vi "_Read Sever Control.vi"(4 "error in (no error)":errorcluster, 5 "Text? (F)":bool, 7 "Control Ref":refnum<vi>) -> (0 "error out":errorcluster, 1 "Text":string, 2 "Boolean":bool)   [LabVIEW 2012]
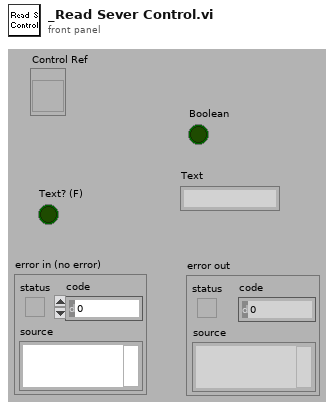
[diagram p1: front panel]
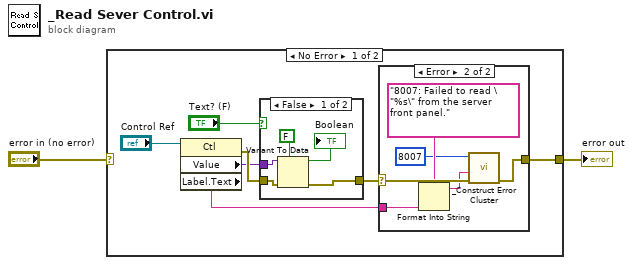
[diagram p0: block diagram]
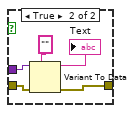
[diagram p3: hidden frame]
diagram:
  n1 = case shown="No Error" "error in (no error)" {
    selector: "error in (no error)" -> [_ w26]
    tunnel: [w9 w26] -> w1
    frame No Error {
      n2 = property class="Ctl"(reference="Control Ref") -> (error out=w7:errorcluster, "Value"=w6:variant, "Label.Text"=w3:string)  [unwired: 1 in, 1 out]
      n3 = case shown="False" "Text? (F)" {
        tunnel: w7 -> [w20 w25]
        tunnel: w6 -> [w19 w24]
        tunnel: [w17 w23] -> w4
        frame False {
          n4 = Variant To Data(error in=w20, type=FALSE, Variant=w19) -> (data=→"Boolean":bool, error out=w17:errorcluster)
        }
        frame True {
          n5 = Variant To Data(error in=w25, type="", Variant=w24) -> (data=→"Text":string, error out=w23:errorcluster)
        }
      }
      n6 = case shown="Error" w4 {
        selector: w4 -> [_ w14]
        tunnel: w3 -> [_ w15]
        tunnel: [_ w11] -> w9
        frame No Error {
        }
        frame Error {
          n7 = Format Into String(format string="8007: Failed to read \"%s\" from the server front panel.", w15) -> (resulting string=w12:string)  [unwired: 2 in, 1 out]
          n8 = call "_Construct Error Cluster.vi"("error in"=w14, "reason"=w12, "errorCode"=8007) -> ("error out"=w11:errorcluster)  [unwired: 1 in, 3 out]
        }
      }
    }
    frame Error {
    }
  }
  "error out" <- w1
